vi "Main_myRIO_v3.1.vi"() -> ()   [LabVIEW 2018]
doc: "Main VI for the controls"
uses:
  components/pmcl dynamic signal analyzer/Controls/DSA excitation specs.ctl
  components/pmcl dynamic signal analyzer/Controls/DSA cycle specs.ctl
  Typedefs/StateDef_Enum.ctl
  <vilib>/Simulation/Scripting/Companion Diagram/SimConfigNode/SimParams.ctl
  <vilib>/Simulation/Scripting/Companion Diagram/SimConfigNode/_simSolvers.ctl
  <vilib>/Simulation/Implementation/Shared/SIMSCR Execution Mode.ctl
  <vilib>/Platform/TimedLoop/XDataNode/timing_clust.ctl
  <vilib>/Platform/TimedLoop/XDataNode/nitl_modes.ctl
  <vilib>/Platform/TimedLoop/XDataNode/wakeup.ctl
  <vilib>/Simulation/Param Hierarchy/Typedefs/SIMPH Param Control Actions.ctl
  <vilib>/Simulation/Implementation/Shared/SIM limit type.ctl
  <vilib>/Simulation/Scripting/Editor Utilities/SIM subVI tag data.ctl
  <vilib>/Simulation/Scripting/Editor Utilities/SIM subVI execution type.ctl
  <vilib>/Simulation/Implementation/Shared/NILVSim_ParamChanged.vi
  <vilib>/Simulation/Implementation/Shared/NILVSim_FinishedLate.vi
  <vilib>/Simulation/Implementation/Shared/NILVSIM_BeginStep.vi
  <vilib>/myRIO/Instrument Drivers/Onboard IO/AI/vis/Read.vi
  <vilib>/Simulation/Utility/Implementation/SIM SimulationParams.vi
  <vilib>/Simulation/ContinuousLinear/Implementation/NILVSim Integrator new.llb/SIM Integrator distributor (scalar).vi
  <vilib>/Simulation/Implementation/Shared/SIM Fire Discrete SubVI.vi
  <vilib>/Simulation/ContinuousLinear/Implementation/NILVSim Transfer Function Direct.llb/SIM Transfer Function Direct (SISO).vi
  <vilib>/Simulation/Utility/Implementation/SIM Halt.vi
  <vilib>/Simulation/SignalArithmetic/Implementation/NILVSim Gain.llb/SIM Gain (scalar).vi
  <vilib>/Simulation/ContinuousLinear/Implementation/NILVSim Integrator new.llb/SIM Integrator collector (scalar).vi
  <vilib>/Simulation/Implementation/Shared/NILVSim_Manager.vi
  <vilib>/Utility/error.llb/Clear Errors.vi
  <vilib>/Simulation/Implementation/Shared/NILVSim_FinalizeModel.vi
  <vilib>/Simulation/Utility/Implementation/NILVSim SimulationParams (core).vi
  <vilib>/Simulation/Implementation/Shared/SIM Fire Discrete SubVI (Core).vi
  <vilib>/myRIO/Common/Instrument Driver Framework/myRIO v1.0/AI/vis/myRIO v1.0 Close AI.vi
  <vilib>/myRIO/Common/Instrument Driver Framework/myRIO v1.0/AO/vis/myRIO v1.0 Close AO.vi
  <vilib>/myRIO/Common/Instrument Driver Framework/myRIO v1.0/AI/vis/myRIO v1.0 Unreserve AI.vi
  <vilib>/myRIO/Common/Instrument Driver Framework/myRIO v1.0/AO/vis/myRIO v1.0 Unreserve AO.vi
  <vilib>/myRIO/Common/Instrument Driver Framework/myRIO v1.0/Resource Manager/vis/myRIO v1.0 Unreserve Channel List.vi
  <vilib>/myRIO/Common/Instrument Driver Framework/myRIO v1.0/AI/vis/myRIO v1.0 Build MUX Configuration AI.vi
  <vilib>/myRIO/Common/Instrument Driver Framework/myRIO v1.0/AO/vis/myRIO v1.0 Build MUX Configuration AO.vi
  <vilib>/myRIO/Common/Instrument Driver Framework/myRIO v1.0/Resource Manager/vis/myRIO v1.0 Unreserve Channel.vi
  <vilib>/myRIO/Common/Instrument Driver Framework/myRIO v1.0/Resource Manager/vis/myRIO v1.0 Build Mutex Name.vi
  <vilib>/Simulation/Implementation/Shared/SIM Unbundle Sim Info.vi
  <vilib>/Simulation/Implementation/Shared/SIMSH Read Queue.vi
  <vilib>/Simulation/Implementation/Shared/NILVSim_Initialize.vi
  <vilib>/Utility/error.llb/Error Cluster From Error Code.vi
  <vilib>/myRIO/Common/Instrument Driver Framework/myRIO v1.0/AI/vis/myRIO v1.0 Read AI.vi
  <vilib>/myRIO/Common/Instrument Driver Framework/myRIO v1.0/AO/vis/myRIO v1.0 Write AO.vi
  <vilib>/Simulation/Utility/Implementation/NILVSim Get Time and IsAcceptedStep.vi
  <vilib>/Simulation/Implementation/Shared/NILVSim_GetModelError.vi
  <vilib>/Simulation/Implementation/Shared/SIM Bundle Sim Info.vi
  <vilib>/myRIO/Common/Instrument Driver Framework/Utilities/vis/Configuration Manager.vi
  <vilib>/myRIO/Common/Instrument Driver Framework/Utilities/vis/IO Manager.vi
  <vilib>/myRIO/Common/Instrument Driver Framework/myRIO v1.0/myRIO v1.0 Close.vi
  <vilib>/Simulation/Scripting/Companion Diagram/SimConfigNode/SimDog.xnode
  <vilib>/Platform/TimedLoop/XDataNode/XDataNode.xnode
  <vilib>/Simulation/Implementation/XNodeFramework/SimXNode/SimX.xnode
  Components/Timing/Timing.lvlib
  <vilib>/myRIO/Instrument Drivers/Onboard IO/AI/AI.lvlib
  <vilib>/myRIO/Instrument Drivers/Onboard IO/AO/AO.lvlib
  <vilib>/Platform/TimedLoop/XDataNode/XDNodeRunTimeDep.lvlib
  <vilib>/Analysis/NI_AALPro.lvlib
  <vilib>/ptbypt/NI_PtbyPt.lvlib
  <vilib>/Simulation/ContinuousLinear/Implementation/NILVSim Integrator new.llb/SIM Integrator (scalar).vi
  <vilib>/Simulation/Implementation/Shared/NI_SIM_Implementation.lvlib
panel:
  in  "System Stop Button":bool
  in  "Pause chart?":bool
  in  "Controller Params":enum32{"Page 1"}(tab)
  in  "Kp":dbl=1.0 min=0.0
  in  "Controller On?":bool
  out "Status":string
  in  "Ref. Gen.":enum32{"Analog In", "Manual", "Wave Gen", "DSA"}(tab)=enum."Wave Gen"
  in  "Ref. cmd.":dbl(slide) step=1.0 scale=-10.0..10.0 scale format="%#.1f"
  in  "Signal Cluster":T1={"phase"=0.0, "amplitude"=1.0, "frequency"=1.0, "offset"=1.0, "Signal"=enum."Square"} {"offset" format="%0.2f"; "frequency" format="%0.2f"; "amplitude" format="%0.2f"; "phase" format="%0.2f"}
  in  "Frequency\nResponse":enum16{"Plant", "RR", "CL"}(ring)
  out "DSA \nRunning?":bool
  in  "Stop \nDSA":bool
  in  "Start \nDSA":bool
  in  "DSA excitation specs":T2={"Initial Freq. [Hz]"=10.0, "Final Freq. [Hz]"=999.0, "# pts. in interval"=50, "Samping Time [s]"=0.001, "Amplitude [V]"=1.0, "Offset [V]"=0.0, "Freq Units (F: rad/s, T: Hz)"=TRUE}
  in  "Cycle Specs":T3={"Cycles To \nSettle (M)"=5, "Cycles To \nCalculate (N)"=10}
  in  "Loop Timing":enum32{"CD&Sim", "Ref. gen", "UI"}(tab)
  out "# Finished\nLate counter":dbl
  in  "CD&Sim\nLoop Rate (Hz)":dbl=2000.0 format="%#_4p"
  out "# Finished\nLate counter":dbl
  in  "Ref. Gen.\nLoop Rate (Hz)":dbl=2000.0 format="%#_4p"
  in  "UI Loop rate (Hz)":dbl=1000.0 format="%#_6p"
  in  "Display Waveforms":enum32{"Controller Signals", "DSA "}(tab)
  out "Control Effort":dbl(graph)
  out "Waveform Chart":cluster{"Double":dbl, "Numeric":dbl}(graph)
  out "Phase Bode Plot":cluster{dbl[], dbl[]}(graph)
  out "Magnitude Bode Plot":cluster{dbl[], dbl[]}(graph)
  out "DSA Signals":cluster{"Double":dbl, "Double":dbl}(graph)
  # "Connect the Reference Signal \nto C/AI 1 of the myRIO."
  # "Pinout Config.:\nPort C/AI0 : Plant output being read           by the myRIO.\nPort C/AI1 : Reference signal for the control loop.\nPort C/AO0 : Control effort signal to the plant."
  # "Control Loop Timing"
  # "Ref.  Gen. Loop Timing"
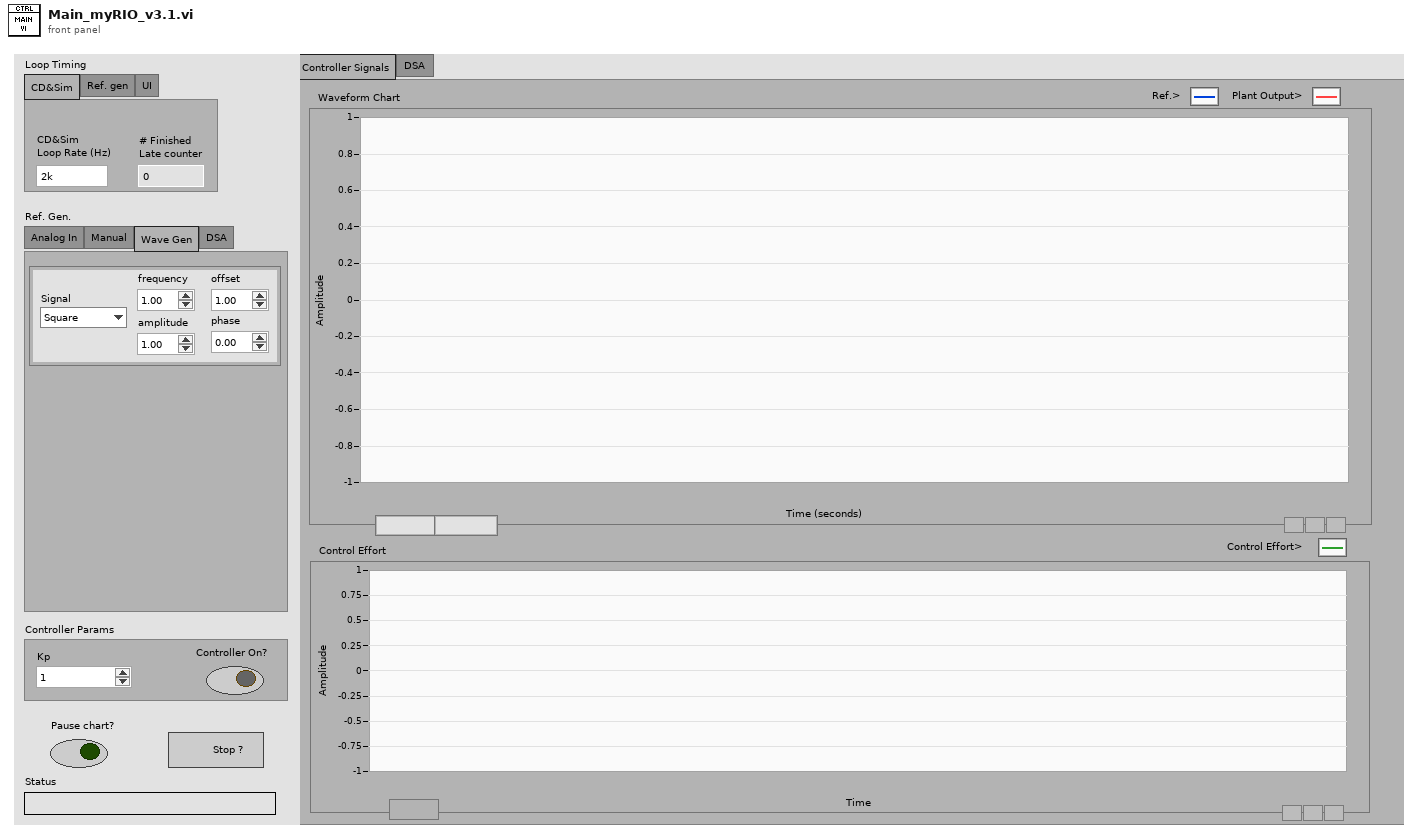
[diagram p1: front panel]
types:
  T1 = cluster{"phase":dbl, "amplitude":dbl, "frequency":dbl, "offset":dbl, "Signal":enum16{"Sine", "Square", "Sawtooth"}}
  T2 = typedef "DSA excitation specs.ctl" = cluster{"Initial Freq. [Hz]":dbl, "Final Freq. [Hz]":dbl, "# pts. in interval":i16, "Samping Time [s]":dbl, "Amplitude [V]":dbl, "Offset [V]":dbl, "Freq Units (F: rad/s, T: Hz)":bool}
  T3 = typedef "DSA cycle specs.ctl" = cluster{"Cycles To \nSettle (M)":i16, "Cycles To \nCalculate (N)":i16}
  T4 = typedef "StateDef_Enum.ctl" = enum16{"Initialize", "Wait", "Shutdown"}
  T5 = typedef "XDNodeRunTimeDep.lvlib/timing_clust.ctl" = cluster{"Expected End [f-1]":u64, "Actual End [f-1]":u64, "Finished Late? [f-1]":bool, "Expected End [i-1]":u64, "Actual End [i-1]":u64, "Finished Late? [i-1]":bool, "Expected Start [i]":u64, "Actual Start [i]":u64, "Expected Start [f]":u64, "Actual Start [f]":u64, "Source Name":string, "Structure Name":string, "Period":i64, "Deadline":i64, "Offset":i64, "Start":i64, "Priority":i32, "Timeout":i32, "Mode":T6, "Wakeup Reason":T7, "Error":errorcluster, "Source Type":string, "Secondary Source Type":string, "Global End Time":u64, "Global Start Time":u64, "Frame Duration":u64, "Iteration Duration":u64, "Assigned CPU":i32, "I/O Scan Engine Mode":u32}
  T6 = typedef "XDNodeRunTimeDep.lvlib/nitl_modes.ctl" = enum32{"No Change", "Process missed periods, maintain original phase", "Discard missed periods, maintain original phase", "Process missed periods, ignore original phase", "Discard missed periods, ignore original phase"}
  T7 = typedef "XDNodeRunTimeDep.lvlib/wakeup.ctl" = enum32{"Normal", "Aborted", "Asynchronous wakeup", "Timing source error", "Timed loop error", "Timeout"}
  T8 = typedef "AI.lvlib/AI Reference.ctl" = cluster{"myRIO Reference":T9, "AI Channels List":T13, "AI Scaling Constants List":T15}
  T9 = typedef "myRIO Generic Hardware Reference.ctl" = cluster{"myRIO Model":T10, "myRIO Hardware Reference":T11}
  T10 = typedef "Hardware Version Enum.ctl" = enum16{"Unknown", "myRIO-1900", "myRIO-1950", "roboRIO", "NI ELVIS RIO CM", "ELVIS III"}
  T11 = typedef "myRIO v1.0 Reference.ctl" = cluster{"Generic FPGA Reference":T12, "Allow multiple opens":bool}
  T12 = typedef "Generic FPGA Reference.ctl" = refnum<k20>
  T13 = typedef "AI Channels List.ctl" = T14[]
  T14 = typedef "AI Channels Enum.ctl" = enum16{"Not Connected", "AudioIn/Left", "AudioIn/Right", "C/AI0", "C/AI1", "A/AI0", "A/AI1", "A/AI2", "A/AI3", "A/AI4", "A/AI5", "A/AI6", "A/AI7", "B/AI0", "B/AI1", "B/AI2", "B/AI3", "B/AI4", "B/AI5", "B/AI6", "B/AI7", "AI/AI0", "AI/AI1", "AI/AI2", "AI/AI3", "A/AI0 (DIFF)", "A/AI1 (DIFF)", "A/AI2 (DIFF)", "A/AI3 (DIFF)", "B/AI0 (DIFF)", "B/AI1 (DIFF)", "B/AI2 (DIFF)", "B/AI3 (DIFF)"}
  T15 = typedef "Analog Scaling Constants List.ctl" = T16[]
  T16 = typedef "Analog Scaling Constants.ctl" = cluster{"LSB Weight (Volts)":dbl, "Offset (Volts)":dbl, "Signed?":bool}
  T17 = typedef "AO.lvlib/AO Reference.ctl" = cluster{"myRIO Reference":T9, "AO Channel List":T18, "AO Scaling Constant List":T15}
  T18 = typedef "AO Channels List.ctl" = T19[]
  T19 = typedef "AO Channels Enum.ctl" = enum16{"Not Connected", "AudioOut/Left", "AudioOut/Right", "C/AO0", "C/AO1", "A/AO0", "A/AO1", "B/AO0", "B/AO1"}
  T20 = cluster{"Analog In CH1":dbl, "Analog In CH0":dbl}
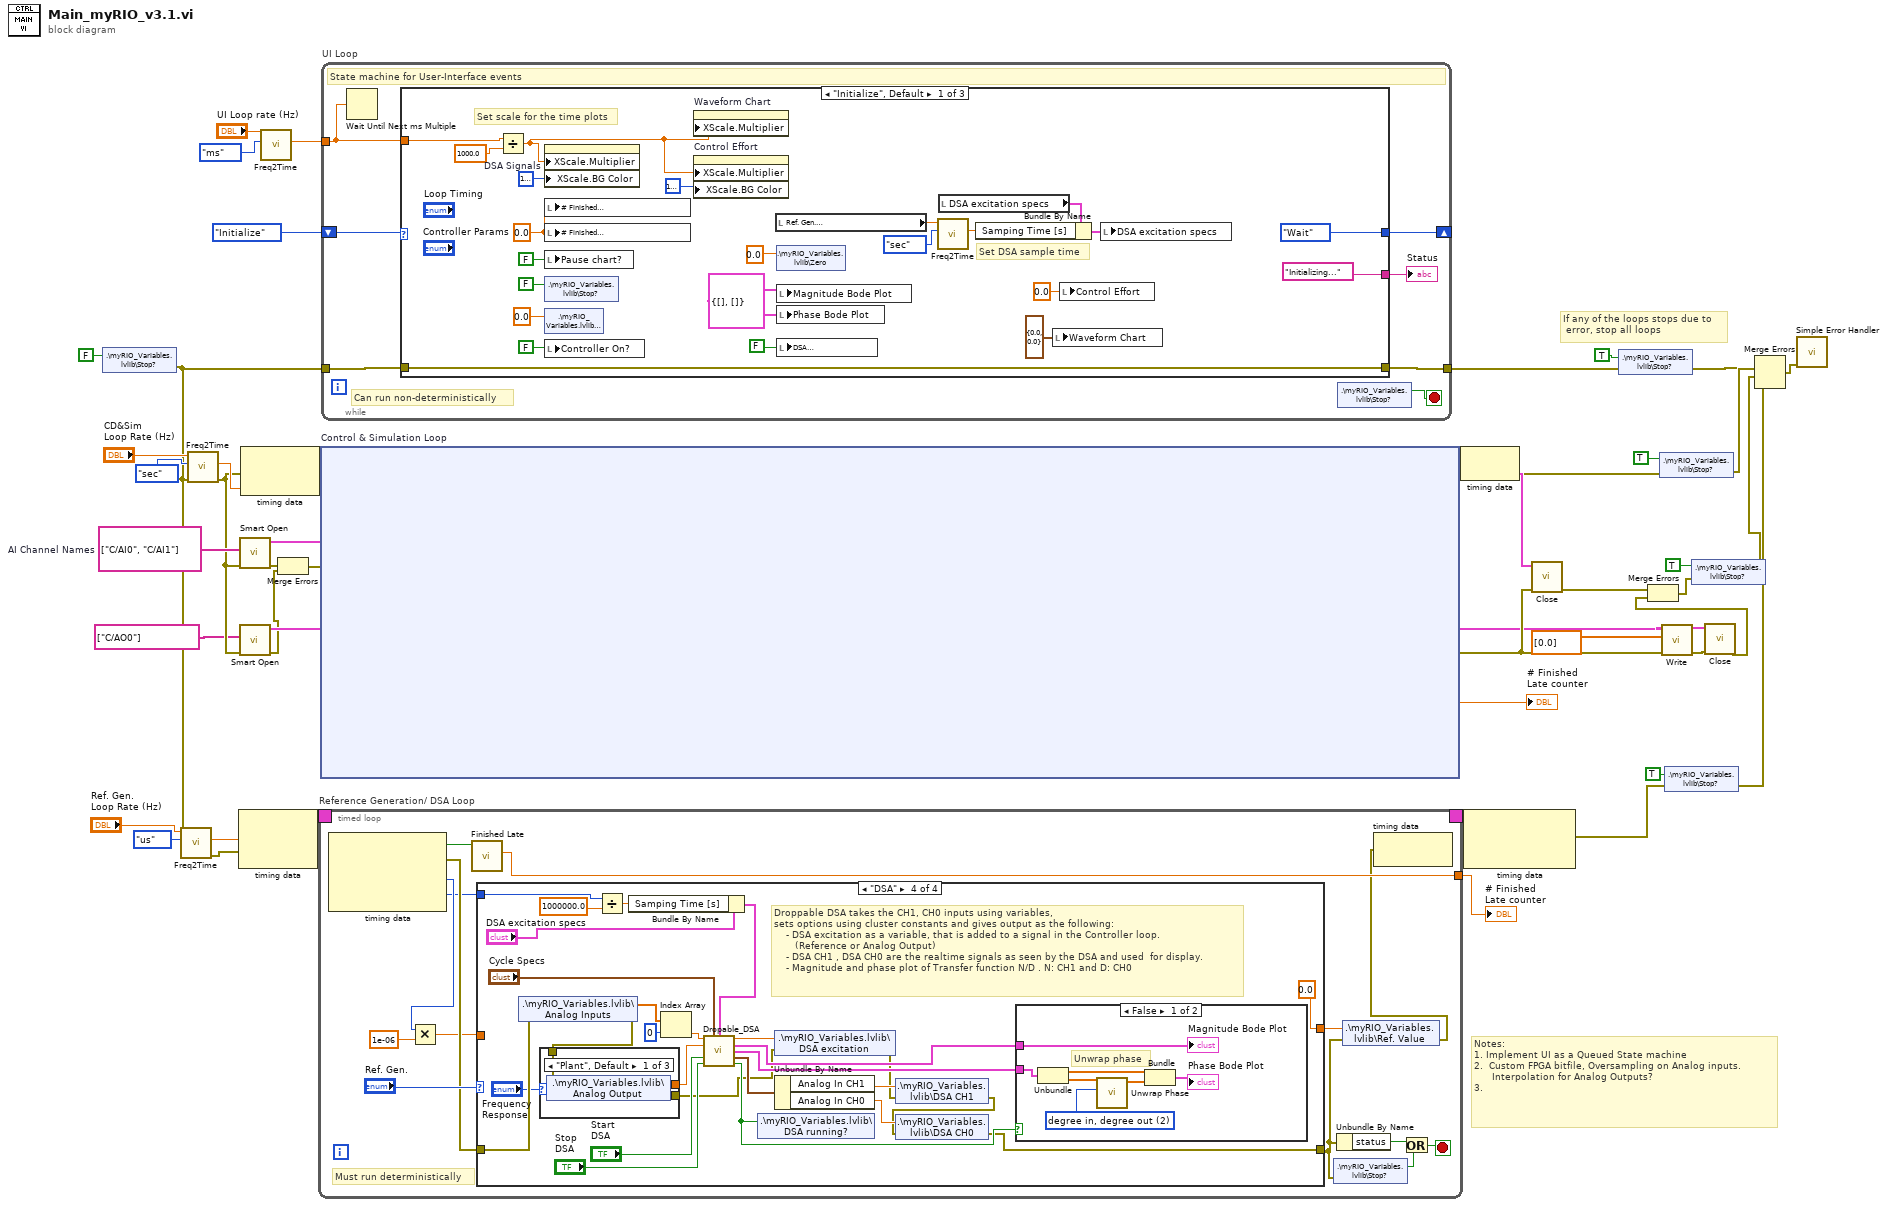
[diagram p0: block diagram]
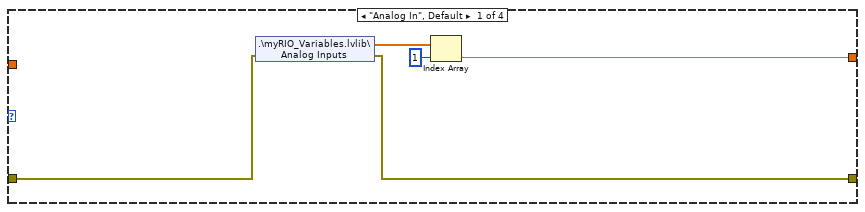
[diagram p2: hidden frame]
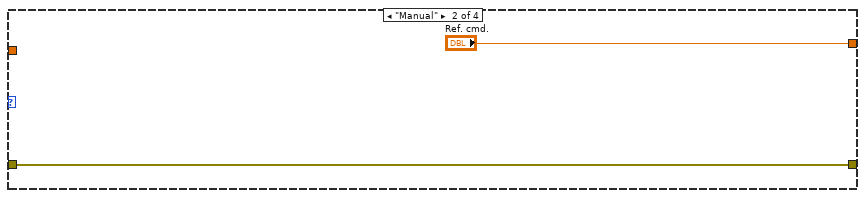
[diagram p3: hidden frame]
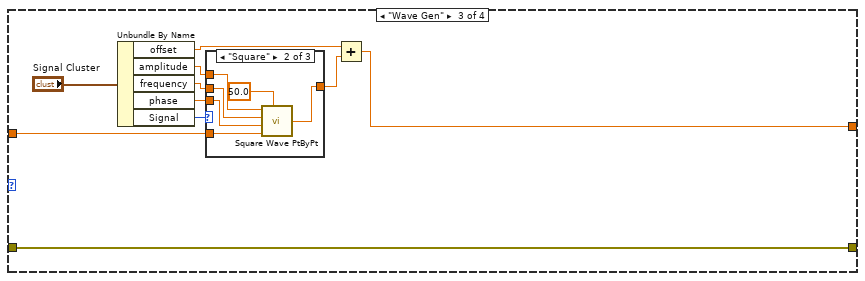
[diagram p4: hidden frame]
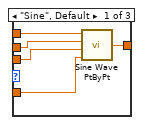
[diagram p5: hidden frame]
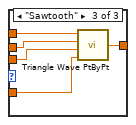
[diagram p6: hidden frame]
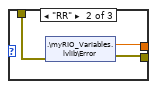
[diagram p7: hidden frame]
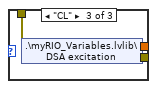
[diagram p8: hidden frame]
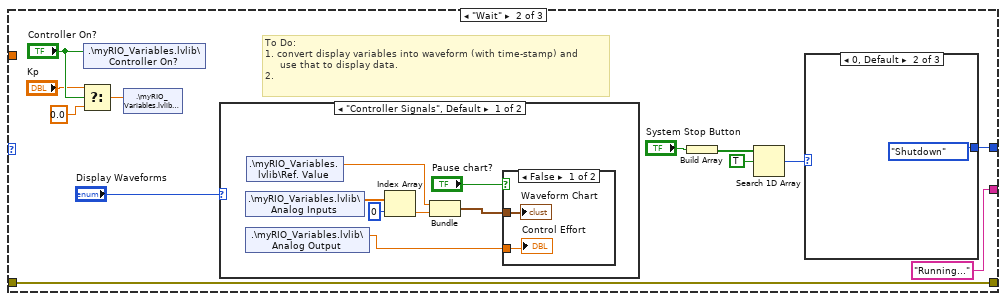
[diagram p10: hidden frame]
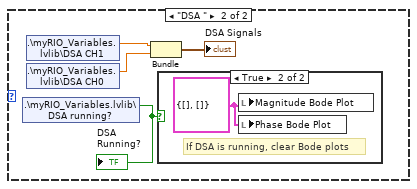
[diagram p12: hidden frame]
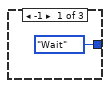
[diagram p14: hidden frame]
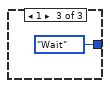
[diagram p15: hidden frame]
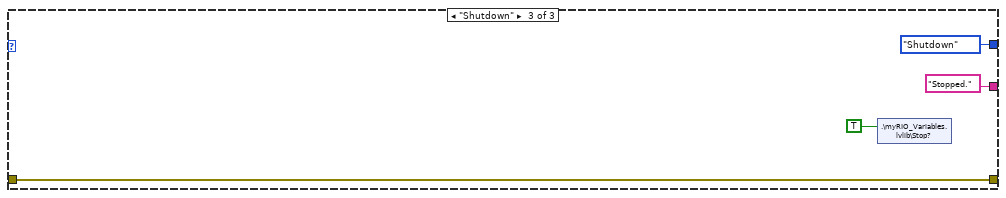
[diagram p16: hidden frame]
diagram:
  w38 = tag[] ["C/AI0", "C/AI1"]  # AI Channel Names
  # "Notes:\n1. Implement UI as a Queued State machine\n2.  Custom FPGA bitfile, Oversampling on Analog inputs. \n      Interpolation for Analog Outputs?\n3."
  # "If any of the loops stops due to\n error, stop all loops"
  n1 = shared-variable ".\\myRIO_Variables.lvlib\\Stop?"(FALSE ("Stop?")) -> (error out=w4:errorcluster)  [unwired: 1 in]
  n2 = call "Freq2Time.vi"("error in (no error)"=w4, "Int. Time Unit"=enum16{"sec", "us", "ms"}."us", "Sample rate (Hz)"="Ref. Gen.\nLoop Rate (Hz)") -> ("error out"=w24:errorcluster, "Int.  time [unit]"=w28:dbl)  [unwired: 6 in, 1 out]
  n3 = call "Freq2Time.vi"("error in (no error)"=w4, "Int. Time Unit"=enum16{"sec", "us", "ms"}."sec", "Sample rate (Hz)"="CD&Sim\nLoop Rate (Hz)") -> ("error out"=w25:errorcluster, "Int.  time [unit]"=w43:dbl)  [unwired: 6 in, 1 out]
  n4 = node-c288(w28, w24) -> (w31:T5)
  n5 = call <vilib>:"Smart Open.vi"("error in (no error)"=w25, "Channel Names"=w38) -> ("error out"=w39:errorcluster, "AI Ref Out"=w40:T8)  [unwired: 8 in]
  n6 = call <vilib>:"Smart Open.vi"("error in (no error)"=w25, "Channel Names"=tag[] ["C/AO0"]) -> ("error out"=w35:errorcluster, "AO Ref Out"=w37:T17)  [unwired: 8 in]
  n7 = node-c288(w25, w43) -> (w47:variant)
  n8 = call "Freq2Time.vi"("Int. Time Unit"=enum16{"sec", "us", "ms"}."ms", "Sample rate (Hz)"="UI Loop rate (Hz)") -> ("Int.  time [unit]"=w9:dbl)  [unwired: 7 in, 2 out]
  n9 = Merge Errors(w39, w35) -> (w36:errorcluster)
  n10 = timed-loop "Reference Generation/ DSA Loop" {
    timing: w31 -> [_]
    timing-out: [_] -> w30
    tunnel: [w61] -> w26
    stop <- w55 stop-if-true
    # "Must run deterministically"
    n11 = node-c288() -> (w62:bool, w58:errorcluster, w52:i64, w51:i64)  [unwired: 1 in]
    n12 = Multiply(x=w52, y=1e-06) -> (x*y=w54:dbl)
    n13 = call "Finished Late.vi"("Finished \nLate?"=w62) -> ("# Finished\nLate counter"=w61:dbl)  [unwired: 8 in, 2 out]
    n14 = case shown="\"DSA\"" "Ref. Gen." {
      tunnel: [w67 "Ref. cmd." w72 0.0 ("Ref. cmd.")] -> w59
      tunnel: w58 -> [w65 w68 w71 w102]
      tunnel: [w64 w68 w71 w105] -> w49
      tunnel: w54 -> [_ _ w70 _]
      tunnel: w51 -> [_ _ _ w112]
      frame "Analog In", Default {
        n15 = shared-variable ".\\myRIO_Variables.lvlib\\Analog Inputs"(error in=w65) -> (w66:dbl[], error out=w64:errorcluster)
        n16 = Index Array(array=w66, index=1) -> (element=w67:dbl)
      }
      frame "Manual" {
      }
      frame "Wave Gen" {
        n17 = Unbundle By Name("Signal Cluster") -> ("offset"=w73:dbl, "amplitude"=w76:dbl, "frequency"=w75:dbl, "phase"=w74:dbl, "Signal"=w77:enum16{"Sine", "Square", "Sawtooth"})
        n18 = case shown="\"Square\"" w77 {
          tunnel: [w84 w89 w95] -> w79
          tunnel: w76 -> [w83 w88 w94]
          tunnel: w75 -> [w82 w87 w93]
          tunnel: w74 -> [w81 w86 w92]
          tunnel: w70 -> [w80 w85 w91]
          frame "Sine", Default {
            n19 = call <vilib>:"Sine Wave PtByPt.vi"("time"=w80, "phase"=w81, "frequency"=w82, "amplitude"=w83) -> ("sine wave"=w84:dbl)
          }
          frame "Square" {
            n20 = call <vilib>:"Square Wave PtByPt.vi"("amplitude"=w88, "frequency"=w87, "phase"=w86, "time"=w85, "duty cycle (%)"=50.0) -> ("square wave"=w89:dbl)
          }
          frame "Sawtooth" {
            n21 = call <vilib>:"Triangle Wave PtByPt.vi"("time"=w91, "phase"=w92, "frequency"=w93, "amplitude"=w94) -> ("triangle wave"=w95:dbl)
          }
        }
        n22 = Add(x=w73, y=w79) -> (x+y=w72:dbl)
      }
      frame "DSA" {
        # "Droppable DSA takes the CH1, CH0 inputs using variables, \nsets options using cluster constants and gives output as the following:\n    - DSA excitation as a variable, that is added to a signal in the Controller loop. \n       (Reference or Analog Output)\n    - DSA CH1 , DSA CH0 are the realtime signals as seen by the DSA and used  for display.\n    - Magnitude and phase plot of Transfer function N/D . N: CH1 and D: CH0"
        n23 = shared-variable ".\\myRIO_Variables.lvlib\\Analog Inputs"(error in=w102) -> (w101:dbl[], error out=w99:errorcluster)
        n24 = case shown="\"Plant\", Default" "Frequency\nResponse" {
          tunnel: [w125 w128 w129] -> w100
          tunnel: w99 -> [w124 w126 w131]
          tunnel: [w123 w127 w130] -> w96
          frame "Plant", Default {
            n25 = shared-variable ".\\myRIO_Variables.lvlib\\Analog Output"(error in=w124) -> (w125:dbl, error out=w123:errorcluster)
          }
          frame "RR" {
            n26 = shared-variable ".\\myRIO_Variables.lvlib\\Error"(error in=w126) -> (w128:dbl, error out=w127:errorcluster)
          }
          frame "CL" {
            n27 = shared-variable ".\\myRIO_Variables.lvlib\\DSA excitation"(error in=w131) -> (w129:dbl, error out=w130:errorcluster)
          }
        }
        n28 = Divide(x=w112, y=1000000.0) -> (x/y=w110:dbl)
        n29 = Bundle By Name(cluster="DSA excitation specs", "Samping Time [s]"=w110) -> (w109:T2)
        n30 = Index Array(array=w101, index=0) -> (element=w103:dbl)
        n31 = call "Dropable_DSA.vi"("Analog In CH1"=w103, "Cycle Specs"="Cycle Specs", "Excitation Specs"=w109, "Analog In CH0"=w100, "START"="Start \nDSA", "STOP"="Stop \nDSA") -> ("Analog Out"=w121:dbl, "Bode Magnitude"=w114:cluster{dbl[], dbl[]}, "Bode Phase"=w113:cluster{dbl[], dbl[]}, "Live signals"=w118:T20, "Running"=w108:bool)  [unwired: 4 in, 1 out]
        n32 = shared-variable ".\\myRIO_Variables.lvlib\\DSA running?"(w108) -> ()  [unwired: 1 in, 1 out]
        n33 = shared-variable ".\\myRIO_Variables.lvlib\\DSA excitation"(w121, error in=w96) -> (error out=w107:errorcluster)
        n34 = Unbundle By Name(w118) -> ("Analog In CH1"=w117:dbl, "Analog In CH0"=w116:dbl)
        n35 = shared-variable ".\\myRIO_Variables.lvlib\\DSA CH1"(w117, error in=w107) -> (error out=w106:errorcluster)
        n36 = shared-variable ".\\myRIO_Variables.lvlib\\DSA CH0"(w116, error in=w106) -> (error out=w105:errorcluster)
        n37 = case shown="False" w108 {
          tunnel: w114 -> [w132 _]
          tunnel: w113 -> [w134 _]
          frame False {
            w136 = 2 items=["radian in, radian out", "radian in, degree out", "degree in, degree out", "degree in, radian out"] ("phase unit")
            # "Unwrap phase"
            n38 = Unbundle(w134) -> (w138:dbl[], w135:dbl[])
            n39 = call <vilib>:"Unwrap Phase.vi"("phase unit"=w136, "Phase"=w135) -> ("Unwrapped Phase"=w137:dbl[])  [unwired: 8 in, 1 out]
            n40 = Bundle(w138, "Unwrapped Phase"=w137) -> (→"Phase Bode Plot":cluster{dbl[], "Unwrapped Phase":dbl[]})  [unwired: 1 in]
            "Magnitude Bode Plot" <- w132
          }
          frame True {
          }
        }
      }
    }
    n41 = shared-variable ".\\myRIO_Variables.lvlib\\Stop?"(error in=w49) -> (w56:bool)  [unwired: 1 out]
    n42 = Unbundle By Name(w49) -> ("status"=w57:bool)
    n43 = shared-variable ".\\myRIO_Variables.lvlib\\Ref. Value"(w59, error in=w49) -> (error out=w50:errorcluster)
    n44 = node-c288(w50) -> ()  [unwired: 1 out]
    n45 = Or(x=w57, y=w56) -> (x .or. y?=w55:bool)
  }
  "# Finished\nLate counter" <- w26
  n46 = node-c254 "Control & Simulation Loop"(w47, w40, w36, w37) -> (w46:variant, →"# Finished\nLate counter":dbl, w14:T17, w17:errorcluster, w34:T8)
  n47 = while "UI Loop" {
    shift-right: [w152] -> _
    shift-left: StateDef_Enum."Initialize" ("State defining Enum") -> [w153]
    tunnel: w4 -> [w151]
    tunnel: [w150] -> w8
    tunnel: w9 -> [w147]
    stop <- w148 stop-if-true
    # "Can run non-deterministically"
    # "State machine for User-Interface events"
    n48 = Wait Until Next ms Multiple(millisecond multiple=w147) -> ()  [unwired: 1 out]
    n49 = case shown="\"Initialize\", Default" w153 {
      tunnel: [StateDef_Enum."Wait" ("State defining Enum") w185 StateDef_Enum."Shutdown" ("State defining Enum")] -> w152
      tunnel: w151 -> [w173 w183 w209]
      tunnel: [w173 w183 w209] -> w150
      tunnel: ["Initializing..." ("Status") "Running..." ("Status") "Stopped." ("Status")] -> w149
      tunnel: w147 -> [w171 _ _]
      frame "Initialize", Default {
        w165 = cluster{dbl[], dbl[]} {[], []} ("Magnitude Bode Plot")
        w167 = 0.0 ("# Finished\nLate counter")
        # "Set DSA sample time"
        # "Set scale for the time plots"
        n50 = Divide(x=w171, y=1000.0) -> (x/y=w157:dbl)
        n51 = property on="DSA Signals" class="WFChart (strict)"("XScale.Multiplier"=w157, "XScale.BG Color"=u32 16777216) -> ()  [unwired: 2 in, 2 out]
        n52 = local write "# Finished\nLate counter"(w167) -> ()
        n53 = local write "# Finished\nLate counter"(w167) -> ()
        n54 = local write "Pause chart?"(FALSE ("Pause chart?")) -> ()
        n55 = shared-variable ".\\myRIO_Variables.lvlib\\Stop?"(FALSE ("Stop?")) -> ()  [unwired: 1 in, 1 out]
        n56 = shared-variable ".\\myRIO_Variables.lvlib\\Kp"(0.0 ("Kp")) -> ()  [unwired: 1 in, 1 out]
        n57 = local write "Controller On?"(FALSE ("Controller On?")) -> ()
        n58 = property on="Waveform Chart" class="WFChart (strict)"("XScale.Multiplier"=w157) -> ()  [unwired: 2 in, 2 out]
        n59 = property on="Control Effort" class="WFChart (strict)"("XScale.Multiplier"=w157, "XScale.BG Color"=u32 16777216) -> ()  [unwired: 2 in, 2 out]
        n60 = local read "Ref. Gen.\nLoop Rate (Hz)"() -> (w160:dbl)
        n61 = shared-variable ".\\myRIO_Variables.lvlib\\Zero"(0.0 ("Zero")) -> ()  [unwired: 1 in, 1 out]
        n62 = local write "Magnitude Bode Plot"(w165) -> ()
        n63 = local write "Phase Bode Plot"(w165) -> ()
        n64 = local write "DSA \nRunning?"(FALSE ("DSA \nRunning?")) -> ()
        n65 = call "Freq2Time.vi"("Int. Time Unit"=enum16{"sec", "us", "ms"}."sec", "Sample rate (Hz)"=w160) -> ("Int.  time [unit]"=w158:dbl)  [unwired: 7 in, 2 out]
        n66 = local read "DSA excitation specs"() -> (w162:T2)
        n67 = Bundle By Name(cluster=w162, "Samping Time [s]"=w158) -> (w161:T2)
        n68 = local write "Waveform Chart"(cluster{"Double":dbl, "Numeric":dbl} {"Double"=0.0, "Numeric"=0.0} ("Waveform Chart")) -> ()
        n69 = local write "Control Effort"(0.0 ("Control Effort")) -> ()
        n70 = local write "DSA excitation specs"(w161) -> ()
      }
      frame "Wait" {
        # "To Do:\n1. convert display variables into waveform (with time-stamp) and\n     use that to display data.\n2."
        n71 = Select(t="Kp", s="Controller On?", f=0.0) -> (s? t:f=w181:dbl)
        n72 = shared-variable ".\\myRIO_Variables.lvlib\\Controller On?"("Controller On?") -> ()  [unwired: 1 in, 1 out]
        n73 = shared-variable ".\\myRIO_Variables.lvlib\\Kp"(w181) -> ()  [unwired: 1 in, 1 out]
        n74 = case shown="\"Controller Signals\", Default" "Display Waveforms" {
          frame "Controller Signals", Default {
            n75 = shared-variable ".\\myRIO_Variables.lvlib\\Analog Inputs"() -> (w195:dbl[])  [unwired: 1 in, 1 out]
            n76 = shared-variable ".\\myRIO_Variables.lvlib\\Analog Output"() -> (w189:dbl)  [unwired: 1 in, 1 out]
            n77 = shared-variable ".\\myRIO_Variables.lvlib\\Ref. Value"() -> (w192:dbl)  [unwired: 1 in, 1 out]
            n78 = Index Array(array=w195, index=0) -> (element=w194:dbl)
            n79 = Bundle("Double"=w192, "Numeric"=w194) -> (w190:cluster{"Double":dbl, "Numeric":dbl})  [unwired: 1 in]
            n80 = case shown="False" "Pause chart?" {
              tunnel: w190 -> [w197 _]
              tunnel: w189 -> [w196 _]
              frame False {
                "Waveform Chart" <- w197
                "Control Effort" <- w196
              }
              frame True {
              }
            }
          }
          frame "DSA " {
            n81 = shared-variable ".\\myRIO_Variables.lvlib\\DSA running?"() -> (w198:bool)  [unwired: 1 in, 1 out]
            "DSA \nRunning?" <- w198
            n82 = shared-variable ".\\myRIO_Variables.lvlib\\DSA CH1"() -> (w200:dbl)  [unwired: 1 in, 1 out]
            n83 = shared-variable ".\\myRIO_Variables.lvlib\\DSA CH0"() -> (w199:dbl)  [unwired: 1 in, 1 out]
            n84 = Bundle("Double"=w200, "Double"=w199) -> (→"DSA Signals":cluster{"Double":dbl, "Double":dbl})  [unwired: 1 in]
            n85 = case shown="True" w198 {
              frame False {
              }
              frame True {
                w202 = cluster{dbl[], dbl[]} {[], []} ("Magnitude Bode Plot")
                # "If DSA is running, clear Bode plots"
                n86 = local write "Magnitude Bode Plot"(w202) -> ()
                n87 = local write "Phase Bode Plot"(w202) -> ()
              }
            }
          }
        }
        n88 = Build Array("System Stop Button") -> (w187:bool[])
        n89 = Search 1D Array(1D array=w187, element=TRUE) -> (index of element=w184:i32)  [unwired: 1 in]
        n90 = case shown="0, Default" w184 {
          tunnel: [StateDef_Enum."Wait" ("State defining Enum") StateDef_Enum."Shutdown" ("State defining Enum") StateDef_Enum."Wait" ("State defining Enum")] -> w185
          frame -1 {
          }
          frame 0, Default {
          }
          frame 1 {
          }
        }
      }
      frame "Shutdown" {
        n91 = shared-variable ".\\myRIO_Variables.lvlib\\Stop?"(TRUE) -> ()  [unwired: 1 in, 1 out]
      }
    }
    "Status" <- w149
    n92 = shared-variable ".\\myRIO_Variables.lvlib\\Stop?"() -> (w148:bool)  [unwired: 1 in, 1 out]
  }
  n93 = node-c288(w46) -> (w23:errorcluster)
  n94 = node-c288(w30) -> (w20:errorcluster)  [unwired: 1 out]
  n95 = call <vilib>:"Close.vi"("error in (no error)"=w17, "AI Ref In"=w34) -> ("error out"=w33:errorcluster)  [unwired: 9 in]
  n96 = shared-variable ".\\myRIO_Variables.lvlib\\Stop?"(TRUE ("Stop?"), error in=w8) -> (error out=w7:errorcluster)
  n97 = shared-variable ".\\myRIO_Variables.lvlib\\Stop?"(TRUE ("Stop?"), error in=w23) -> (error out=w22:errorcluster)
  n98 = call <vilib>:"Write.vi"("error in (no error)"=w17, "Values"=dbl[] [0.0], "AO Ref In"=w14) -> ("error out"=w16:errorcluster, "AO Ref Out"=w15:T17)  [unwired: 6 in]
  n99 = shared-variable ".\\myRIO_Variables.lvlib\\Stop?"(TRUE ("Stop?"), error in=w20) -> (error out=w19:errorcluster)
  n100 = call <vilib>:"Close.vi"("error in (no error)"=w16, "AO Ref In"=w15) -> ("error out"=w32:errorcluster)  [unwired: 9 in]
  n101 = Merge Errors(w33, w32) -> (w2:errorcluster)
  n102 = shared-variable ".\\myRIO_Variables.lvlib\\Stop?"(TRUE ("Stop?"), error in=w2) -> (error out=w1:errorcluster)
  n103 = Merge Errors(w7, w22, w1, w19) -> (w41:errorcluster)
  n104 = call <vilib>:"Simple Error Handler.vi"("error in (no error)"=w41) -> ()  [unwired: 4 in, 5 out]
